vi "ATSh_ForceTrigger.vi"(11 "Handle":u32) -> (0 "Return Code":u32, 3 "Handle_Out":u32)   [LabVIEW 2015]
doc: "_____AlazarTech, Scope_____\n\nForce the Device to perform a software trigger.\nHandle input."
uses:
  ATSApi.dll
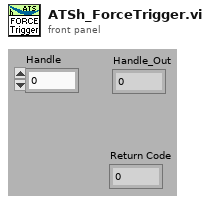
[diagram p1: front panel]
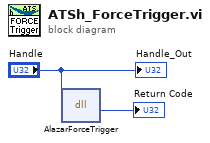
[diagram p0: block diagram]
diagram:
  n1 = dll-call lib="C:/IntensityOCT/trunk/ATSApi.dll" fn="AlazarForceTrigger"("h"="Handle") -> (→"Return Code":u32)  [unwired: 4 in, 2 out]
  "Handle_Out" <- "Handle"
